vi "OSI OPC Client.vi"() -> ()   [LabVIEW 2018]
uses:
  <vilib>/OPCUA/controls/NodeId.ctl
  <vilib>/OPCUA/controls/Node Class.ctl
  <vilib>/OPCUA/controls/Subscription Data Change.ctl
  <vilib>/OPCUA/controls/Data Type.ctl
  <vilib>/OPCUA/controls/OPC UA StatusCode.ctl
  <vilib>/OPCUA/NI OPC UA Client.lvlib
panel:
  out "data change":T1[](array[typedef]) {"data type" items=["Boolean"=1, "SByte"=2, "Byte"=3, "Int16"=4, "UInt16"=5, "Int32"=6, "UInt32"=7, "Int64"=8, "UInt64"=9, "Float"=10, "Double"=11, "String"=12, "DateTime"=13, "ByteString"=15, "Array of Boolean"=101, "Array of SByte"=102, "Array of Byte"=103, "Array of Int16"=104, "Array of UInt16"=105, "Array of Int32"=106, "Array of UInt32"=107, "Array of Int64"=108, "Array of UInt64"=109, "Array of Float"=110, "Array of Double"=111, "Array of String"=112, "Array of DateTime"=113, "Array of ByteString"=115, "Matrix of Boolean"=201, "Matrix of SByte"=202, "Matrix of Byte"=203, "Matrix of Int16"=204, "Matrix of UInt16"=205, "Matrix of Int32"=206, "Matrix of UInt32"=207, "Matrix of Int64"=208, "Matrix of UInt64"=209, "Matrix of Float"=210, "Matrix of Double"=211, "Matrix of String "=212, "Matrix of DateTime"=213, "Matrix of ByteString"=215]; "status code" items=["Good"=0, "Good_SubscriptionTransferred"=2949120, "Good_CompletesAsynchronously"=3014656, "Good_Overload"=3080192, "Good_Clamped"=3145728, "Good_LocalOverride"=9830400, "Good_EntryInserted"=10616832, "Good_EntryReplaced"=10682368, "Good_NoData"=10813440, "Good_MoreData"=10878976, "Good_CommunicationEvent"=10944512, "Good_ShutdownEvent"=11010048, "Good_CallAgain"=11075584, "Good_NonCriticalTimeout"=11141120, "Good_ResultsMayBeIncomplete"=12189696, "Good_DataIgnored"=14221312, "Uncertain"=1073741824, "Uncertain_ReferenceOutOfServer"=1080819712, "Uncertain_NoCommunicationLastUsableValue"=1083113472, "Uncertain_LastUsableValue"=1083179008, "Uncertain_SubstituteValue"=1083244544, "Uncertain_InitialValue"=1083310080, "Uncertain_SensorNotAccurate"=1083375616, "Uncertain_EngineeringUnitsExceeded"=1083441152, "Uncertain_SubNormal"=1083506688, "Uncertain_DataSubNormal"=1084489728, "Uncertain_ReferenceNotDeleted"=1086062592, "Uncertain_NotAllNodesAvailable"=1086324736, "Bad"=2147483648, "Bad_UnexpectedError"=2147549184, "Bad_InternalError"=2147614720, "Bad_OutOfMemory"=2147680256, "Bad_ResourceUnavailable"=2147745792, "Bad_CommunicationError"=2147811328, "Bad_EncodingError"=2147876864, "Bad_DecodingError"=2147942400, "Bad_EncodingLimitsExceeded"=2148007936, "Bad_UnknownResponse"=2148073472, "Bad_Timeout"=2148139008, "Bad_ServiceUnsupported"=2148204544, "Bad_Shutdown"=2148270080, "Bad_ServerNotConnected"=2148335616, "Bad_ServerHalted"=2148401152, "Bad_NothingToDo"=2148466688, "Bad_TooManyOperations"=2148532224, "Bad_DataTypeIdUnknown"=2148597760, "Bad_CertificateInvalid"=2148663296, "Bad_SecurityChecksFailed"=2148728832, "Bad_CertificateTimeInvalid"=2148794368, "Bad_CertificateIssuerTimeInvalid"=2148859904, "Bad_CertificateHostNameInvalid"=2148925440, "Bad_CertificateUriInvalid"=2148990976, "Bad_CertificateUseNotAllowed"=2149056512, "Bad_CertificateIssuerUseNotAllowed"=2149122048, "Bad_CertificateUntrusted"=2149187584, "Bad_CertificateRevocationUnknown"=2149253120, "Bad_CertificateIssuerRevocationUnknown"=2149318656, "Bad_CertificateRevoked"=2149384192, "Bad_CertificateIssuerRevoked"=2149449728, "Bad_UserAccessDenied"=2149515264, "Bad_IdentityTokenInvalid"=2149580800, "Bad_IdentityTokenRejected"=2149646336, "Bad_SecureChannelIdInvalid"=2149711872, "Bad_InvalidTimestamp"=2149777408, "Bad_NonceInvalid"=2149842944, "Bad_SessionIdInvalid"=2149908480, "Bad_SessionClosed"=2149974016, "Bad_SessionNotActivated"=2150039552, "Bad_SubscriptionIdInvalid"=2150105088, "Bad_RequestHeaderInvalid"=2150236160, "Bad_TimestampsToReturnInvalid"=2150301696, "Bad_RequestCancelledByClient"=2150367232, "Bad_NoCommunication"=2150694912, "Bad_WaitingForInitialData"=2150760448, "Bad_NodeIdInvalid"=2150825984, "Bad_NodeIdUnknown"=2150891520, "Bad_AttributeIdInvalid"=2150957056, "Bad_IndexRangeInvalid"=2151022592, "Bad_IndexRangeNoData"=2151088128, "Bad_DataEncodingInvalid"=2151153664, "Bad_DataEncodingUnsupported"=2151219200, "Bad_NotReadable"=2151284736, "Bad_NotWritable"=2151350272, "Bad_OutOfRange"=2151415808, "Bad_NotSupported"=2151481344, "Bad_NotFound"=2151546880, "Bad_ObjectDeleted"=2151612416, "Bad_NotImplemented"=2151677952, "Bad_MonitoringModeInvalid"=2151743488, "Bad_MonitoredItemIdInvalid"=2151809024, "Bad_MonitoredItemFilterInvalid"=2151874560, "Bad_MonitoredItemFilterUnsupported"=2151940096, "Bad_FilterNotAllowed"=2152005632, "Bad_StructureMissing"=2152071168, "Bad_EventFilterInvalid"=2152136704, "Bad_ContentFilterInvalid"=2152202240, "Bad_FilterOperandInvalid"=2152267776, "Bad_ContinuationPointInvalid"=2152333312, "Bad_NoContinuationPoints"=2152398848, "Bad_ReferenceTypeIdInvalid"=2152464384, "Bad_BrowseDirectionInvalid"=2152529920, "Bad_NodeNotInView"=2152595456, "Bad_ServerUriInvalid"=2152660992, "Bad_ServerNameMissing"=2152726528, "Bad_DiscoveryUrlMissing"=2152792064, "Bad_SempahoreFileMissing"=2152857600, "Bad_RequestTypeInvalid"=2152923136, "Bad_SecurityModeRejected"=2152988672, "Bad_SecurityPolicyRejected"=2153054208, "Bad_TooManySessions"=2153119744, "Bad_UserSignatureInvalid"=2153185280, "Bad_ApplicationSignatureInvalid"=2153250816, "Bad_NoValidCertificates"=2153316352, "Bad_RequestCancelledByRequest"=2153381888, "Bad_ParentNodeIdInvalid"=2153447424, "Bad_ReferenceNotAllowed"=2153512960, "Bad_NodeIdRejected"=2153578496, "Bad_NodeIdExists"=2153644032, "Bad_NodeClassInvalid"=2153709568, "Bad_BrowseNameInvalid"=2153775104, "Bad_BrowseNameDuplicated"=2153840640, "Bad_NodeAttributesInvalid"=2153906176, "Bad_TypeDefinitionInvalid"=2153971712, "Bad_SourceNodeIdInvalid"=2154037248, "Bad_TargetNodeIdInvalid"=2154102784, "Bad_DuplicateReferenceNotAllowed"=2154168320, "Bad_InvalidSelfReference"=2154233856, "Bad_ReferenceLocalOnly"=2154299392, "Bad_NoDeleteRights"=2154364928, "Bad_ServerIndexInvalid"=2154430464, "Bad_ViewIdUnknown"=2154496000, "Bad_TooManyMatches"=2154627072, "Bad_QueryTooComplex"=2154692608, "Bad_NoMatch"=2154758144, "Bad_MaxAgeInvalid"=2154823680, "Bad_HistoryOperationInvalid"=2154889216, "Bad_HistoryOperationUnsupported"=2154954752, "Bad_WriteNotSupported"=2155020288, "Bad_TypeMismatch"=2155085824, "Bad_MethodInvalid"=2155151360, "Bad_ArgumentsMissing"=2155216896, "Bad_TooManySubscriptions"=2155282432, "Bad_TooManyPublishRequests"=2155347968, "Bad_NoSubscription"=2155413504, "Bad_SequenceNumberUnknown"=2155479040, "Bad_MessageNotAvailable"=2155544576, "Bad_InsufficientClientProfile"=2155610112, "Bad_TcpServerTooBusy"=2155675648, "Bad_TcpMessageTypeInvalid"=2155741184, "Bad_TcpSecureChannelUnknown"=2155806720, "Bad_TcpMessageTooLarge"=2155872256, "Bad_TcpNotEnoughResources"=2155937792, "Bad_TcpInternalError"=2156003328, "Bad_TcpEndpointUrlInvalid"=2156068864, "Bad_RequestInterrupted"=2156134400, "Bad_RequestTimeout"=2156199936, "Bad_SecureChannelClosed"=2156265472, "Bad_SecureChannelTokenUnknown"=2156331008, "Bad_SequenceNumberInvalid"=2156396544, "Bad_ConfigurationError"=2156462080, "Bad_NotConnected"=2156527616, "Bad_DeviceFailure"=2156593152, "Bad_SensorFailure"=2156658688, "Bad_OutOfService"=2156724224, "Bad_DeadbandFilterInvalid"=2156789760, "Bad_RefreshInProgress"=2157379584, "Bad_ConditionAlreadyDisabled"=2157445120, "Bad_ConditionDisabled"=2157510656, "Bad_EventIdUnknown"=2157576192, "Bad_NoData"=2157641728, "Bad_DataLost"=2157772800, "Bad_DataUnavailable"=2157838336, "Bad_EntryExists"=2157903872, "Bad_NoEntryExists"=2157969408, "Bad_TimestampNotSupported"=2158034944, "Bad_InvalidArgument"=2158690304, "Bad_ConnectionRejected"=2158755840, "Bad_Disconnect"=2158821376, "Bad_ConnectionClosed"=2158886912, "Bad_InvalidState"=2158952448, "Bad_EndOfStream"=2159017984, "Bad_NoDataAvailable"=2159083520, "Bad_WaitingForResponse"=2159149056, "Bad_OperationAbandoned"=2159214592, "Bad_ExpectedStreamToBlock"=2159280128, "Bad_WouldBlock"=2159345664, "Bad_SyntaxError"=2159411200, "Bad_MaxConnectionsReached"=2159476736, "Bad_RequestTooLarge"=2159542272, "Bad_ResponseTooLarge"=2159607808, "Bad_EventNotAcknowledgeable"=2159738880, "Bad_InvalidTimestampArgument"=2159869952, "Bad_ProtocolVersionUnsupported"=2159935488, "Bad_StateNotActive"=2160001024, "Bad_FilterOperatorInvalid"=2160132096, "Bad_FilterOperatorUnsupported"=2160197632, "Bad_FilterOperandCountMismatch"=2160263168, "Bad_FilterElementInvalid"=2160328704, "Bad_FilterLiteralInvalid"=2160394240, "Bad_IdentityChangeNotSupported"=2160459776, "Bad_NotTypeDefinition"=2160590848, "Bad_ViewTimestampInvalid"=2160656384, "Bad_ViewParameterMismatch"=2160721920, "Bad_ViewVersionInvalid"=2160787456, "Bad_ConditionAlreadyEnabled"=2160852992, "Bad_DialogNotActive"=2160918528, "Bad_DialogResponseInvalid"=2160984064, "Bad_ConditionBranchAlreadyAcked"=2161049600, "Bad_ConditionBranchAlreadyConfirmed"=2161115136, "Bad_ConditionAlreadyShelved"=2161180672, "Bad_ConditionNotShelved"=2161246208, "Bad_ShelvingTimeOutOfRange"=2161311744, "Bad_AggregateListMismatch"=2161377280, "Bad_AggregateNotSupported"=2161442816, "Bad_AggregateInvalidInputs"=2161508352, "Bad_BoundNotFound"=2161573888, "Bad_BoundNotSupported"=2161639424, "Bad_AggregateConfigurationRejected"=2161770496, "Bad_TooManyMonitoredItems"=2161836032]}
  out "Array 2":T2[](array[typedef])
  out "browse result":T6(array[cluster]) {"node type" items=["Unspecified"=0, "BaseDataType"=24, "BaseObjectType"=58, "FolderType"=61, "BaseVariableType"=62, "BaseDataVariableType"=63, "PropertyType"=68, "DataTypeDescriptionType"=69, "DataTypeDictionaryType"=72, "DataTypeSystemType"=75, "DataTypeEncodingType"=76, "ModellingRuleType"=77, "NamingRuleType"=120, "IdType"=256, "UserTokenType"=303, "ApplicationType"=307, "SecurityTokenRequestType"=315, "EnumeratedTestType"=398, "ScalarTestType"=399, "ArrayTestType"=402, "CompositeTestType"=405, "DeadbandType"=718, "RedundantServerDataType"=853, "SamplingIntervalDiagnosticsDataType"=856, "ServerDiagnosticsSummaryDataType"=859, "ServerStatusDataType"=862, "SessionDiagnosticsDataType"=865, "SessionSecurityDiagnosticsDataType"=868, "ServiceCounterDataType"=871, "SubscriptionDiagnosticsDataType"=874, "ModelChangeStructureDataType"=877, "ProgramDiagnosticDataType"=894, "SemanticChangeStructureDataType"=897, "ServerType"=2004, "ServerCapabilitiesType"=2013, "ServerDiagnosticsType"=2020, "SessionsDiagnosticsSummaryType"=2026, "SessionDiagnosticsObjectType"=2029, "VendorServerInfoType"=2033, "ServerRedundancyType"=2034, "TransparentRedundancyType"=2036, "NonTransparentRedundancyType"=2039, "BaseEventType"=2041, "AuditEventType"=2052, "AuditSecurityEventType"=2058, "AuditChannelEventType"=2059, "AuditOpenSecureChannelEventType"=2060, "AuditSessionEventType"=2069, "AuditCreateSessionEventType"=2071, "AuditActivateSessionEventType"=2075, "AuditCancelEventType"=2078, "AuditCertificateEventType"=2080, "AuditCertificateDataMismatchEventType"=2082, "AuditCertificateExpiredEventType"=2085, "AuditCertificateInvalidEventType"=2086, "AuditCertificateUntrustedEventType"=2087, "AuditCertificateRevokedEventType"=2088, "AuditCertificateMismatchEventType"=2089, "AuditNodeManagementEventType"=2090, "AuditAddNodesEventType"=2091, "AuditDeleteNodesEventType"=2093, "AuditAddReferencesEventType"=2095, "AuditDeleteReferencesEventType"=2097, "AuditUpdateEventType"=2099, "AuditWriteUpdateEventType"=2100, "AuditHistoryUpdateEventType"=2104, "AuditUpdateMethodEventType"=2127, "SystemEventType"=2130, "DeviceFailureEventType"=2131, "BaseModelChangeEventType"=2132, "GeneralModelChangeEventType"=2133, "ServerVendorCapabilityType"=2137, "ServerStatusType"=2138, "ServerDiagnosticsSummaryType"=2150, "SamplingIntervalDiagnosticsArrayType"=2164, "SamplingIntervalDiagnosticsType"=2165, "SubscriptionDiagnosticsArrayType"=2171, "SubscriptionDiagnosticsType"=2172, "SessionDiagnosticsArrayType"=2196, "SessionDiagnosticsVariableType"=2197, "SessionSecurityDiagnosticsArrayType"=2243, "SessionSecurityDiagnosticsType"=2244, "StateMachineType"=2299, "StateType"=2307, "InitialStateType"=2309, "TransitionType"=2310, "TransitionEventType"=2311, "AuditUpdateStateEventType"=2315, "HistoricalDataConfigurationType"=2318, "HistoryServerCapabilitiesType"=2330, "AggregateFunctionType"=2340, "DataItemType"=2365, "AnalogItemType"=2368, "DiscreteItemType"=2372, "TwoStateDiscreteType"=2373, "MultiStateDiscreteType"=2376, "ProgramTransitionEventType"=2378, "ProgramDiagnosticType"=2380, "ProgramStateMachineType"=2391, "SemanticChangeEventType"=2738, "AuditUrlMismatchEventType"=2748, "StateVariableType"=2755, "FiniteStateVariableType"=2760, "TransitionVariableType"=2762, "FiniteTransitionVariableType"=2767, "FiniteStateMachineType"=2771, "ConditionType"=2782, "RefreshStartEventType"=2787, "RefreshEndEventType"=2788, "RefreshRequiredEventType"=2789, "AuditConditionEventType"=2790, "AuditConditionEnableEventType"=2803, "AuditConditionCommentEventType"=2829, "DialogConditionType"=2830, "AcknowledgeableConditionType"=2881, "AlarmConditionType"=2915, "ShelvedStateMachineType"=2929, "LimitAlarmType"=2955, "AuditHistoryEventUpdateEventType"=2999, "AuditHistoryValueUpdateEventType"=3006, "AuditHistoryDeleteEventType"=3012, "AuditHistoryRawModifyDeleteEventType"=3014, "AuditHistoryAtTimeDeleteEventType"=3019, "AuditHistoryEventDeleteEventType"=3022, "EventQueueOverflowEventType"=3035, "BuildInfoType"=3051, "ProgramTransitionAuditEventType"=3806, "EnumValueType"=7594, "TimeZoneDataType"=8912, "LockType"=8921, "AuditConditionRespondEventType"=8927, "AuditConditionAcknowledgeEventType"=8944, "AuditConditionConfirmEventType"=8961, "TwoStateVariableType"=8995, "ConditionVariableType"=9002, "ExclusiveLimitStateMachineType"=9318, "ExclusiveLimitAlarmType"=9341, "ExclusiveLevelAlarmType"=9482, "ExclusiveRateOfChangeAlarmType"=9623, "ExclusiveDeviationAlarmType"=9764, "NonExclusiveLimitAlarmType"=9906, "NonExclusiveLevelAlarmType"=10060, "NonExclusiveRateOfChangeAlarmType"=10214, "NonExclusiveDeviationAlarmType"=10368, "DiscreteAlarmType"=10523, "OffNormalAlarmType"=10637, "TripAlarmType"=10751, "AuditConditionShelvingEventType"=11093, "BaseConditionClassType"=11163, "ProcessConditionClassType"=11164, "MaintenanceConditionClassType"=11165, "SystemConditionClassType"=11166, "AggregateConfigurationType"=11187, "HistoryUpdateType"=11234, "MultiStateValueDiscreteType"=11238, "PerformUpdateType"=11293, "ProgressEventType"=11436, "SystemStatusChangeEventType"=11446, "OptionSetType"=11487, "OperationLimitsType"=11564, "FileType"=11575, "AddressSpaceFileType"=11595, "NamespaceMetadataType"=11616, "NamespacesType"=11645, "BitFieldMaskDataType"=11737, "SystemOffNormalAlarmType"=11753, "AuditProgramTransitionEventType"=11856, "EndpointUrlListDataType"=11943, "NetworkGroupDataType"=11944, "NonTransparentNetworkRedundancyType"=11945, "ArrayItemType"=12021, "YArrayItemType"=12029, "XYArrayItemType"=12038, "ImageItemType"=12047, "CubeItemType"=12057, "NDimensionArrayItemType"=12068, "XVType"=12080, "ComplexNumberType"=12171, "DoubleComplexNumberType"=12172, "TrustListType"=12522, "TrustListDataType"=12554, "CertificateGroupType"=12555, "CertificateType"=12556, "ApplicationCertificateType"=12557, "HttpsCertificateType"=12558, "RsaMinApplicationCertificateType"=12559, "RsaSha256ApplicationCertificateType"=12560, "TrustListUpdatedAuditEventType"=12561, "ServerConfigurationType"=12581, "CertificateUpdatedAuditEventType"=12620, "CertificateExpirationAlarmType"=13225, "FileDirectoryType"=13353, "CertificateGroupFolderType"=13813]; "node class" items=["Unspecified"=0, "Object"=1, "Variable"=2, "Method"=4, "Object Type"=8, "Variable Type"=16, "Reference Type"=32, "Data Type"=64, "View"=128]; "reference type" items=["Unspecified"=0, "Organizes"=35, "Has Event Source"=36, "Has Subtype"=45, "Has Property"=46, "Has Component"=47, "Has Notifier"=48, "Has Ordered Component"=49]}
  out "Array":dbl[](array[numeric])
  in  "security policy":T7={"message mode"=enum."Sign", "security"=enum."Basic256"}
  in  "stop":bool
  in  "server endpoint URL":string="opc.tcp://localhost:49580"
  # "opc.tcp://localhost:49580"
  # "opc.tcp://AMRGROBJ07MYKD:49580"
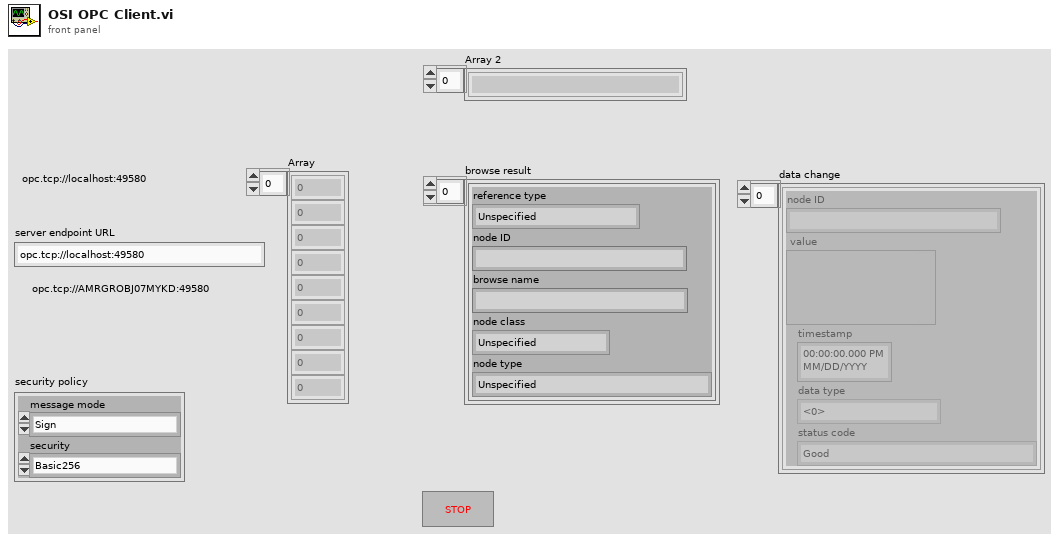
[diagram p1: front panel]
types:
  T1 = typedef "Subscription Data Change.ctl" = cluster{"node ID":T2, " value":variant, "timestamp":timestamp, "data type":T3, "status code":T4}
  T2 = typedef "NodeId.ctl" = string
  T3 = typedef "Data Type.ctl" = u16
  T4 = typedef "OPC UA StatusCode.ctl" = u32
  T5 = typedef "Node Class.ctl" = u32
  T6 = cluster{"reference type":u32, "node ID":T2, "browse name":string, "node class":T5, "node type":u32}[]
  T7 = cluster{"message mode":enum16{"None", "Sign", "Sign and Encrypt"}, "security":enum16{"Basic256", "Basic128Rsa15"}}
  T8 = typedef "OPC UA Client Refnum.ctl" = refnum<k21>
  T9 = typedef "Subscription ID.ctl" = u32
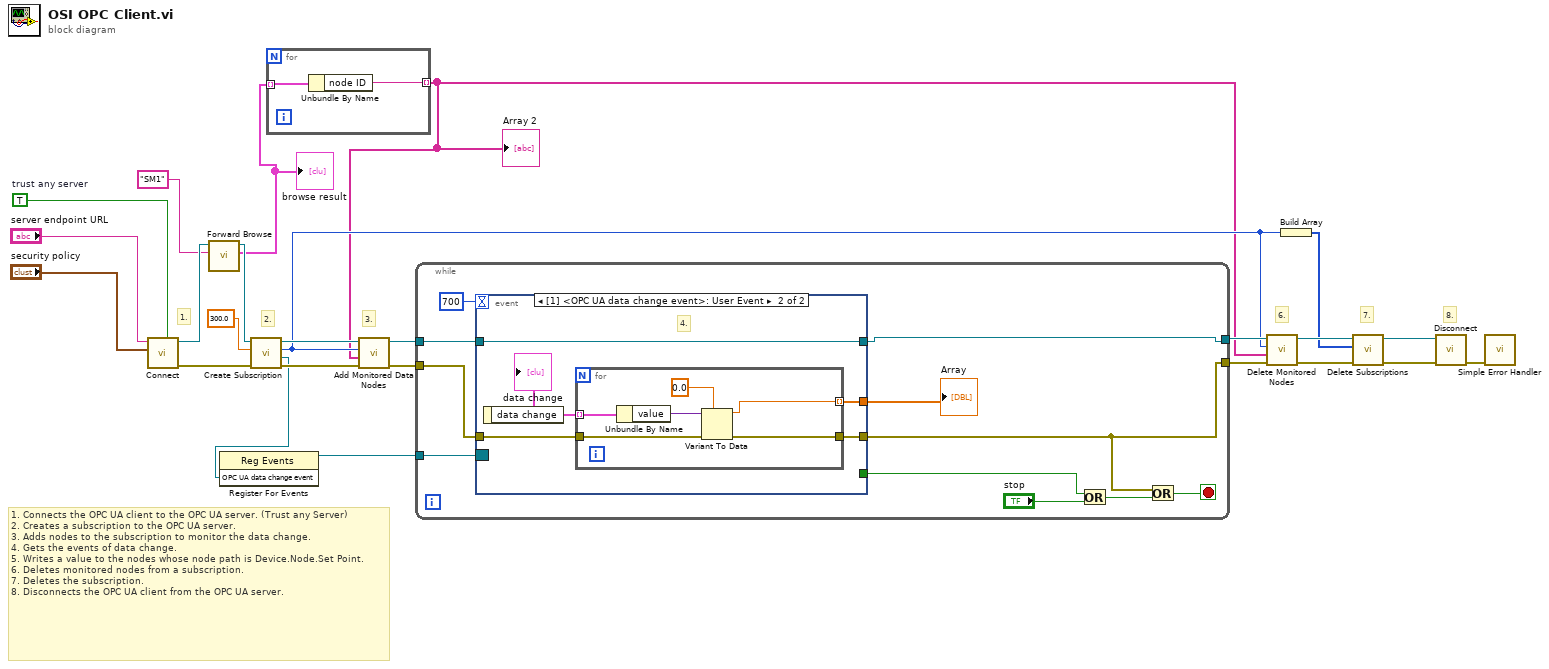
[diagram p0: block diagram]
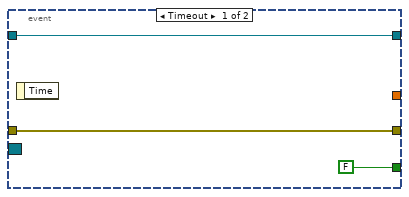
[diagram p2: hidden frame]
diagram:
  w7 = TRUE  # trust any server
  # "7."
  # "1. Connects the OPC UA client to the OPC UA server. (Trust any Server) \n2. Creates a subscription to the OPC UA server.\n3. Adds nodes to the subscription to monitor the data change.\n4. Gets the events of data change.\n5. Writes a value to the nodes whose node path is Device.Node.Set Point. \n6. Deletes monitored nodes from a subscription.\n7. Deletes the subscription.\n8. Disconnects the OPC UA client from the OPC UA server."
  # "8."
  # "6."
  # "3."
  # "2."
  # "1."
  n1 = call <vilib>:"Connect.vi"("trust any server (F)"=w7, "security policy"="security policy", "server endpoint URL"="server endpoint URL") -> ("error out"=w13:errorcluster, "OPC UA client refnum out"=w6:T8)  [unwired: 6 in, 1 out]
  n2 = call <vilib>:"Forward Browse.vi"("node ID"=T2 "SM1", "OPC UA client refnum in"=w6) -> ("browse result"=w3:T6, "OPC UA client refnum out"=w5:T8)  [unwired: 6 in, 2 out]
  "browse result" <- w3
  n3 = call <vilib>:"Create Subscription.vi"("error in (no error)"=w13, "publishing interval (1000 ms)"=300.0 ("update rate (1000 ms)"), "OPC UA client refnum in"=w5) -> ("error out"=w23:errorcluster, "OPC UA data change event"=w1:refnum<user-event>, "subscription ID out"=w11:T9, "OPC UA client refnum out"=w24:T8)  [unwired: 4 in, 1 out]
  n4 = register-events(w1) -> (reference out=w22:refnum<event-registration>)  [unwired: 2 in, 1 out]
  n5 = for {
    tunnel: w3 -> [w27] mode=indexing
    tunnel: [w26] -> w2 mode=indexing
    n6 = Unbundle By Name(w27) -> ("node ID"=w26:T2)
  }
  "Array 2" <- w2
  n7 = call <vilib>:"Add Monitored Data Nodes.vi"("error in (no error)"=w23, "node IDs"=w2, "subscription ID in"=w11, "OPC UA client refnum in"=w24) -> ("error out"=w20:errorcluster, "OPC UA client refnum out"=w21:T8)  [unwired: 4 in, 2 out]
  n8 = while {
    tunnel: w22 -> [w38]
    tunnel: w21 -> [w36]
    tunnel: w20 -> [w34]
    tunnel: [w32] -> w18
    tunnel: [w35] -> w19
    stop <- w33 stop-if-true
    n9 = event shown="[1] <OPC UA data change event>: User Event" {
      selector: w38 -> [_ _]
      dyn-events: _ -> [_ _]
      timeout: 700 -> [_ _]
      tunnel: w36 -> [w41 w43]
      tunnel: [w41 w43] -> w35
      tunnel: [w40 w44] -> w32
      tunnel: w34 -> [w40 w45]
      tunnel: [FALSE _] -> w30
      tunnel: [_ w42] -> w28
      event Timeout {
        n10 = event-data() -> ()  [unwired: 1 in, 1 out]
      }
      event User Event {
        # "4."
        n11 = event-data() -> ("data change"=w46:T1[])  [unwired: 1 in]
        "data change" <- w46
        n12 = for {
          tunnel: w46 -> [w52] mode=indexing
          tunnel: w45 -> [w50]
          tunnel: [w49] -> w44
          tunnel: [w47] -> w42 mode=indexing
          n13 = Unbundle By Name(w52) -> ("value"=w51:variant)
          n14 = Variant To Data(error in=w50, type=0.0, Variant=w51) -> (data=w47:dbl, error out=w49:errorcluster)
        }
      }
    }
    "Array" <- w28
    n15 = Or(x=w30, y="stop") -> (x .or. y?=w29:bool)
    n16 = Or(x=w32, y=w29) -> (x .or. y?=w33:bool)
  }
  n17 = call <vilib>:"Delete Monitored Nodes.vi"("error in (no error)"=w18, "node IDs"=w2, "subscription ID in"=w11, "OPC UA client refnum in"=w19) -> ("error out"=w16:errorcluster, "OPC UA client refnum out"=w17:T8)  [unwired: 3 in, 3 out]
  n18 = Build Array(w11) -> (w10:T9[])
  n19 = call <vilib>:"Delete Subscriptions.vi"("error in (no error)"=w16, "subscription IDs"=w10, "OPC UA client refnum in"=w17) -> ("error out"=w14:errorcluster, "OPC UA client refnum out"=w15:T8)  [unwired: 6 in, 1 out]
  n20 = call <vilib>:"Disconnect.vi"("error in (no error)"=w14, "OPC UA client refnum in"=w15) -> ("error out"=w8:errorcluster)  [unwired: 9 in]
  n21 = call <vilib>:"Simple Error Handler.vi"("error in (no error)"=w8) -> ()  [unwired: 4 in, 5 out]
